vi "Hatch Super Slam TeleOp.vi"(11 "Controller Values":T1) -> ()   [LabVIEW 2018]
uses:
  Support Code/Controller Values.ctl
  <vilib>/Rock Robotics/Network Tables/NT Write Boolean.vi
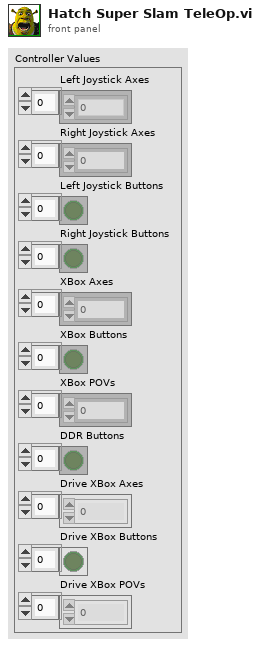
[diagram p1: front panel]
types:
  T1 = typedef "Controller Values.ctl" = cluster{"Left Joystick Axes ":dbl[], "Right Joystick Axes":dbl[], "Left Joystick Buttons":bool[], "Right Joystick Buttons":bool[], "XBox Axes":dbl[], "XBox Buttons":bool[], "XBox POVs":i16[], "DDR Buttons":bool[], "Drive XBox Axes":dbl[], "Drive XBox Buttons":bool[], "Drive XBox POVs":i16[]}
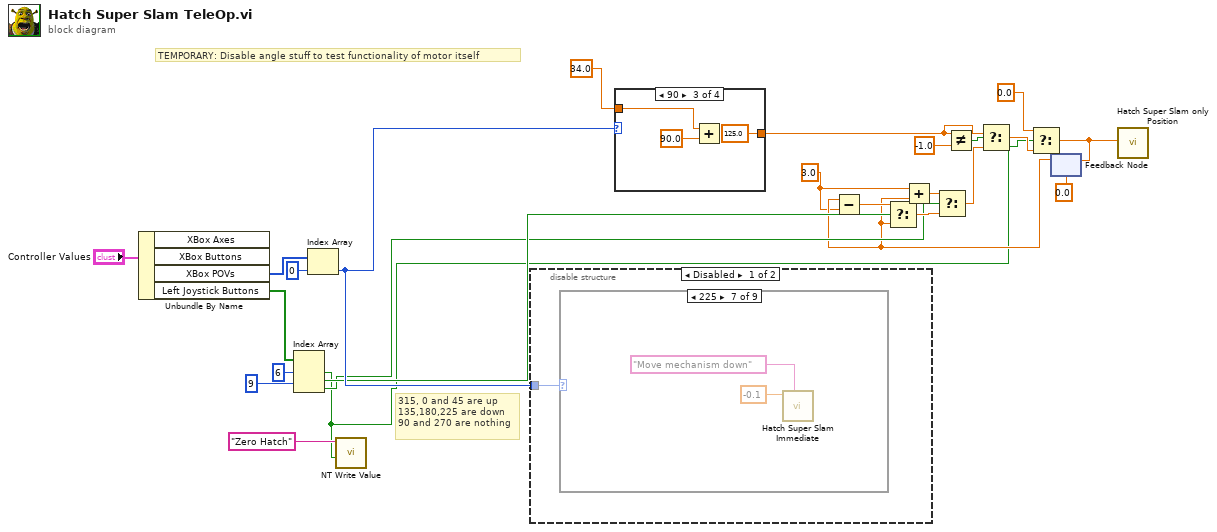
[diagram p0: block diagram]
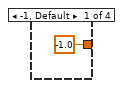
[diagram p2: hidden frame]
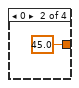
[diagram p3: hidden frame]
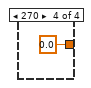
[diagram p4: hidden frame]
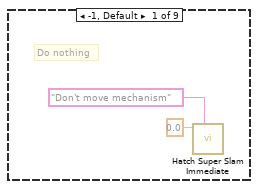
[diagram p5: hidden frame]
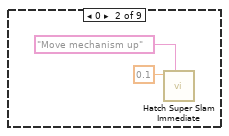
[diagram p6: hidden frame]
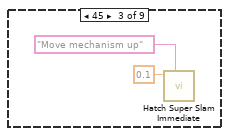
[diagram p7: hidden frame]
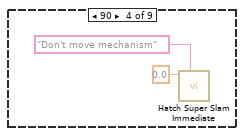
[diagram p8: hidden frame]
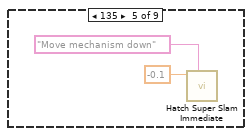
[diagram p9: hidden frame]
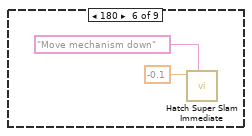
[diagram p10: hidden frame]
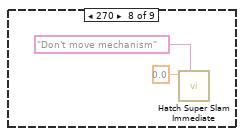
[diagram p11: hidden frame]
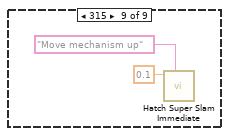
[diagram p12: hidden frame]
diagram:
  w5 = 3.0 ("y")
  # "315, 0 and 45 are up\n135,180,225 are down\n90 and 270 are nothing"
  # "TEMPORARY: Disable angle stuff to test functionality of motor itself"
  n1 = Unbundle By Name("Controller Values") -> ("XBox POVs"=w23:i16[], "Left Joystick Buttons"=w17:bool[])  [unwired: 2 out]
  n2 = Index Array(array=w17, index #1=6 ("index"), index #2=9 ("index")) -> (element #1=w2:bool, element #2=w10:bool, element #3=w9:bool)  [unwired: 1 in]
  n3 = Index Array(array=w23, index=0) -> (element=w20:i16)
  n4 = call-poly <vilib>:"NT Write Value.vi"("Boolean"=w2, "Name"="Zero Hatch") -> ()  [unwired: 9 in, 1 out]
  n5 = disable-structure shown="Disabled" {
    disable-tunnel: w20 -> [w26 _]
    frame Disabled {
      n6 = case shown="225" w26 {
        frame -1, Default {
          # "Do nothing"
          n7 = call "Hatch Super Slam Immediate.vi"("Description"="Don't move mechanism", "Setpoint"=0.0) -> ()  [unwired: 9 in, 1 out]
        }
        frame 0 {
          n8 = call "Hatch Super Slam Immediate.vi"("Description"="Move mechanism up", "Setpoint"=0.1) -> ()  [unwired: 9 in, 1 out]
        }
        frame 45 {
          n9 = call "Hatch Super Slam Immediate.vi"("Description"="Move mechanism up", "Setpoint"=0.1) -> ()  [unwired: 9 in, 1 out]
        }
        frame 90 {
          n10 = call "Hatch Super Slam Immediate.vi"("Description"="Don't move mechanism", "Setpoint"=0.0) -> ()  [unwired: 9 in, 1 out]
        }
        frame 135 {
          n11 = call "Hatch Super Slam Immediate.vi"("Description"="Move mechanism down", "Setpoint"=-0.1) -> ()  [unwired: 9 in, 1 out]
        }
        frame 180 {
          n12 = call "Hatch Super Slam Immediate.vi"("Description"="Move mechanism down", "Setpoint"=-0.1) -> ()  [unwired: 9 in, 1 out]
        }
        frame 225 {
          n13 = call "Hatch Super Slam Immediate.vi"("Description"="Move mechanism down", "Setpoint"=-0.1) -> ()  [unwired: 9 in, 1 out]
        }
        frame 270 {
          n14 = call "Hatch Super Slam Immediate.vi"("Description"="Don't move mechanism", "Setpoint"=0.0) -> ()  [unwired: 9 in, 1 out]
        }
        frame 315 {
          n15 = call "Hatch Super Slam Immediate.vi"("Description"="Move mechanism up", "Setpoint"=0.1) -> ()  [unwired: 9 in, 1 out]
        }
      }
    }
    frame Enabled {
    }
  }
  n16 = case shown="90" w20 {
    tunnel: 34.0 ("Encoder value") -> [_ _ w48 _]
    tunnel: [-1.0 45.0 ("Encoder value") 125.0 ("Encoder value") 0.0] -> w19
    frame -1, Default {
    }
    frame 0 {
    }
    frame 90 {
      n17 = Add(x=w48, y=90.0) -> ()  [unwired: 1 out]
    }
    frame 270 {
    }
  }
  n18 = Not Equal?(x=w19, y=-1.0) -> (x != y?=w22:bool)
  n19 = feedback #1(0.0) -> (w6:dbl)
  n20 = Subtract(x=w6, y=w5) -> (x-y=w8:dbl)
  n21 = Select(t=w8, s=w10, f=w6) -> (s? t:f=w13:dbl)
  n22 = Add(x=w5, y=w6) -> (x+y=w7:dbl)
  n23 = Select(t=w7, s=w9, f=w13) -> (s? t:f=w12:dbl)
  n24 = Select(t=w19, s=w22, f=w12) -> (s? t:f=w3:dbl)
  n25 = Select(t=0.0, s=w2, f=w3) -> (s? t:f=w4:dbl)
  n26 = feedback-in #1(w4) -> ()
  n27 = call "Hatch Super Slam only Position.vi"("Position"=w4) -> ()  [unwired: 10 in, 1 out]
